vi "PH_SHS_Analysis_Calibrator.evt call Select Cam.vi"(0 "i ref in":refnum<vi>, 3 "Cam":string, 5 "error in":errorcluster) -> (14 "i ref out":refnum<vi>, 19 "error out":errorcluster)   [LabVIEW 2014, in "PH_SHS_Analysis_Calibrator.lvlib"]
doc: "This VI calls \"SelectCam\" by a simple call."
uses:
  PH_SHS_Analysis_Calibrator.lvlib
  CS_Core/CSSystem/CoreLib/CoreLib.string 2 byte array.vi
  CS_Core/CSSystem/CSSystemLib/CSSystemLib.lvlib
  CS_Core/CSSystem/CoreLib/CoreLib.lvlib
  CS_Core/BaseProcess/BaseProcess.lvlib
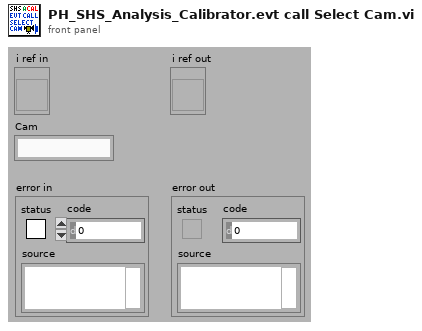
[diagram p1: front panel]
types:
  T1 = typedef "CoreDefs.rawDataType.ctl" = i8[]
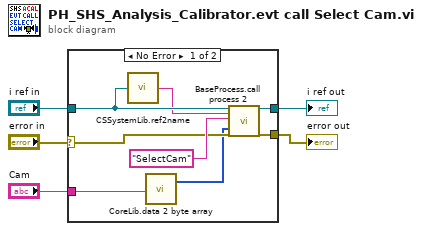
[diagram p0: block diagram]
diagram:
  n1 = case shown="No Error" "error in" {
    selector: "error in" -> [w8 w14]
    tunnel: [w12 w14] -> w5
    tunnel: [w11 w15] -> w4
    tunnel: "Cam" -> [w7 _]
    tunnel: "i ref in" -> [w10 w15]
    frame No Error {
      n2 = call "CSSystemLib.ref2name.vi"("obj refnum"=w10) -> ("name"=w9:string)
      n3 = call-poly "CoreLib.data 2 byte array.vi"("string"=w7) -> ("byteArray out"=w6:T1)  [unwired: 18 in]
      n4 = call "BaseProcess.call process 2.vi"("i ref in"=w10, "Object"=w9, "Selector"="SelectCam", "Data"=w6, "error in (no error)"=w8) -> ("i ref out"=w11:refnum<vi>, "error out"=w12:errorcluster)  [unwired: 13 in]
    }
    frame Error {
    }
  }
  "error out" <- w5
  "i ref out" <- w4
